vi "GetBits_LeCroy.vi"(0 "VISA resource name":refnum<visa-resource-name>, 11 "error in (no error)":errorcluster) -> (4 "VISA resource name out":refnum<visa-resource-name>, 8 "Nom_Bits":i16, 15 "error out":errorcluster)   [LabVIEW 2022 SP3]
doc: "Get basic information about acquisition waveform from specified channel."
uses:
  <instrlib>/LeCroy Wave Series/LeCroy Wave Series.lvlib
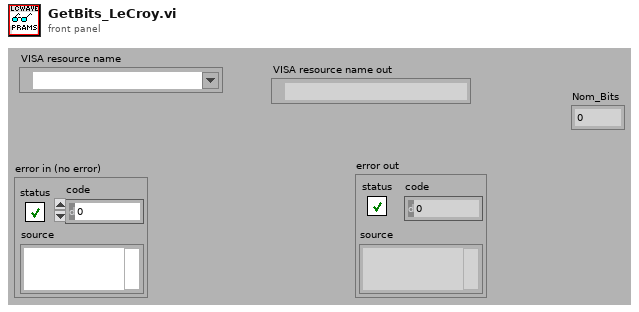
[diagram p1: front panel]
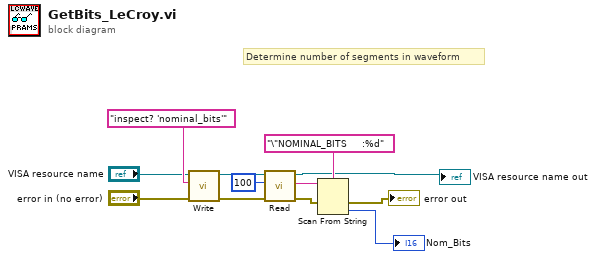
[diagram p0: block diagram]
diagram:
  # "Determine number of segments in waveform"
  n1 = call <instrlib>:"Write.vi"("error in (no error)"="error in (no error)", "Write Buffer"="inspect? 'nominal_bits'", "VISA resource name"="VISA resource name") -> ("error out"=w8:errorcluster, "VISA resource name out"=w6:refnum<visa-resource-name>)  [unwired: 6 in, 1 out]
  n2 = call <instrlib>:"Read.vi"("error in (no error)"=w8, "Byte Count"=u32 100, "VISA resource name"=w6) -> ("error out"=w12:errorcluster, "Read Buffer"=w10:string, "VISA resource name out"=→"VISA resource name out":refnum<visa-resource-name>)  [unwired: 5 in, 1 out]
  n3 = Scan From String(format string="\"NOMINAL_BITS     :%d", input string=w10, error in=w12) -> (error out=→"error out":errorcluster, output 1=→"Nom_Bits":i16)  [unwired: 2 in, 2 out]
